vi "PH_BeamlineController.set wanted Path to World.vi"(0 "VI in":refnum<vi>, 5 "error in (no error)":errorcluster) -> (14 "VI out":refnum<vi>, 19 "error out":errorcluster)   [LabVIEW 2014, in "PH_BeamlineController.lvlib"]
uses:
  PH_BeamlineController.lvlib
  PH_SystemInformation/PH_SystemInformationEnabling State.ctl
  PH_Beamline/PH_Beamline.6P Switch Instances.ctl
  PH_Beamline/PH_Beamline.Black Box Instances.ctl
  PH_StatusHandler/PH_StatusHandler.Status.ctl
  PH_BeamlineController.Targets.ctl
  PH_BeamlineController.PA DP Targets.ctl
  PH_Beamline/PH_Beamline.Switch Instances.ctl
  PH_Beamline/PH_Beamline.lvlib
  PH_BlackBox/PH_BlackBox.lvlib
  PH_SystemInformation/PH_SystemInformation.lvlib
  PH_Sixpack_Switch/PH_Sixpack_Switch.lvlib
  PH_Switch/PH_Switch.lvlib
  PH_StatusHandler/PH_StatusHandler.lvlib
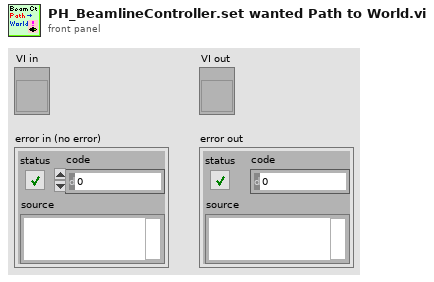
[diagram p1: front panel]
types:
  T1 = typedef "PH_Beamline.lvlib/PH_Beamline.Black Box Instances.ctl" = string
  T2 = typedef "PH_BeamlineController.lvlib/PH_BeamlineController.PA DP Targets.ctl" = enum16{"None", "Dump PA Delayed Beam", "Dump PA Undelayed Beam", "Dumps PA Delayed and Undelayed Beam"}
  T3 = typedef "PH_BeamlineController.lvlib/PH_BeamlineController.Targets.ctl" = enum16{"None", "PreAmp", "Dump Exp Laserlab", "Exp Laserlab", "Calorimeter", "Dump Exp Laserbay", "Exp Laserbay", "Dump Exp Z6", "Exp Z6"}
  T4 = typedef "PH_StatusHandler.lvlib/PH_StatusHandler.Status.ctl" = i16
  T5 = typedef "PH_SystemInformation.lvlib/PH_SystemInformationEnabling State.ctl" = i32
  T6 = enum16{"Laser", "PreAmp", "MainAmp", "Exp 1", "Exp 2", "Exp 3", "Exp 4"}
  T7 = typedef "PH_Beamline.lvlib/PH_Beamline.6P Switch Instances.ctl" = string
  T8 = typedef "PH_BeamlineController.lvlib/PH_BeamlineController.Sources.ctl" = enum16{"None", "YLF", "fs-Frontend", "ns-Frontend", "YLF and ns-Frontend", "fs- and ns-Frontend"}
  T9 = typedef "PH_Beamline.lvlib/PH_Beamline.Switch Instances.ctl" = string
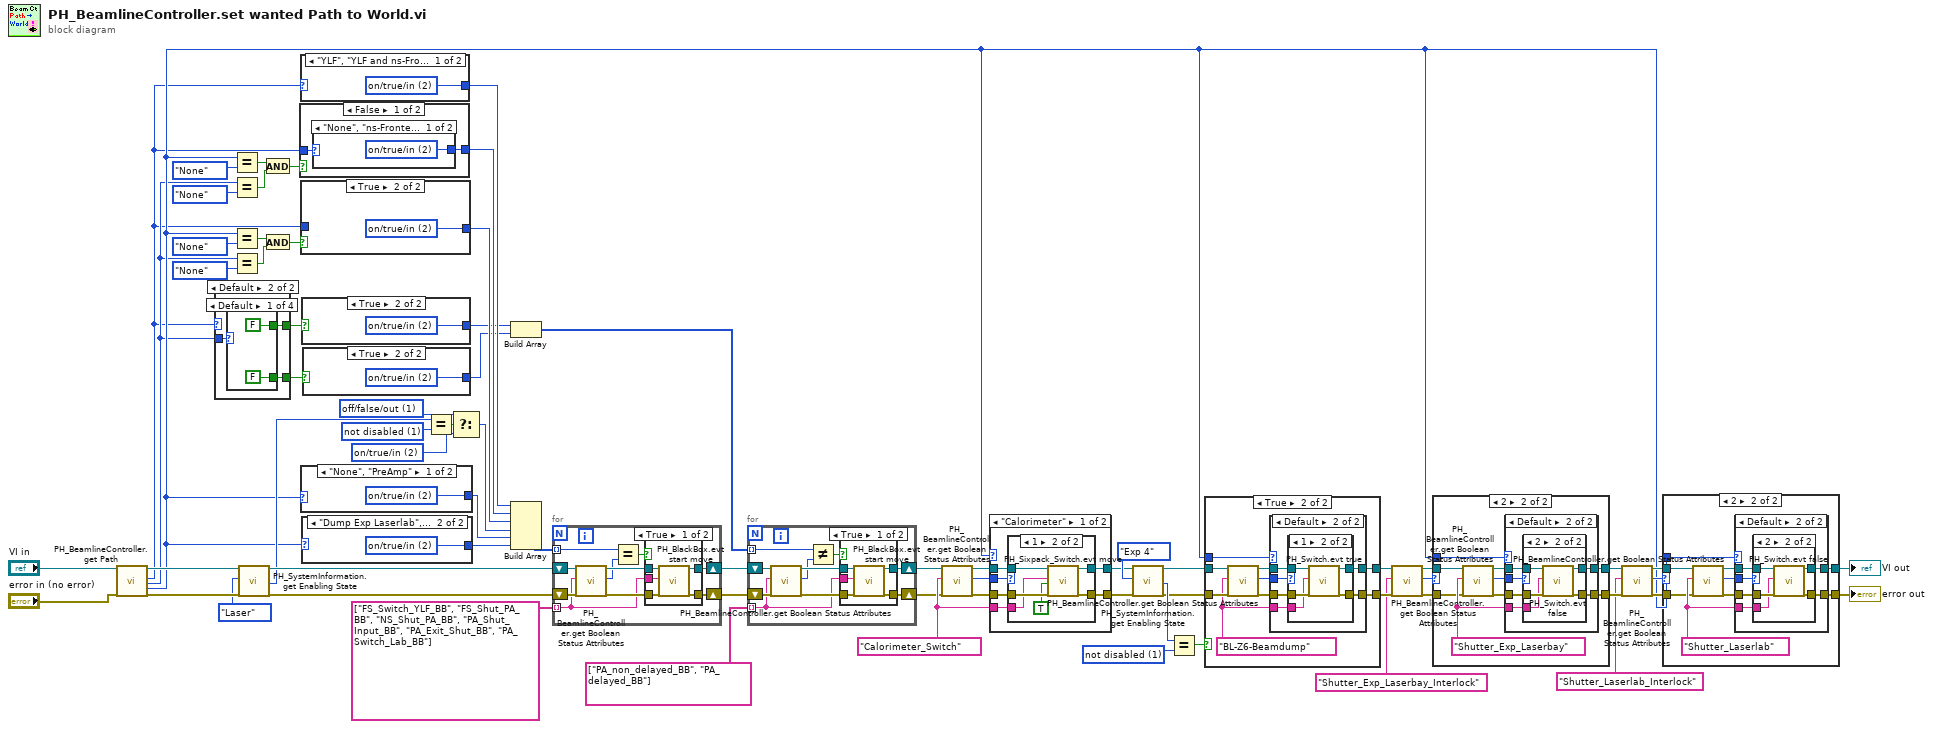
[diagram p0: block diagram]
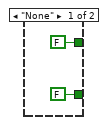
[diagram p3: hidden frame]
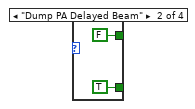
[diagram p4: hidden frame]
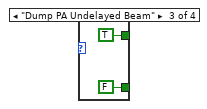
[diagram p5: hidden frame]
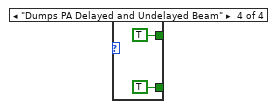
[diagram p6: hidden frame]
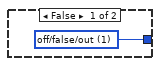
[diagram p7: hidden frame]
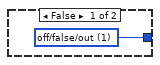
[diagram p8: hidden frame]
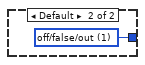
[diagram p10: hidden frame]
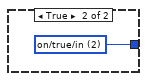
[diagram p11: hidden frame]
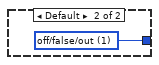
[diagram p12: hidden frame]
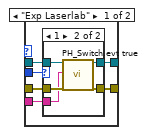
[diagram p14: hidden frame]
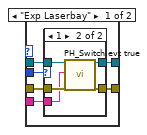
[diagram p18: hidden frame]
diagram:
  w44 = T4 2 items=["no info", "off/false/out", "on/true/in", "Failure", "Alarm", "Status 1", "Status 2", "Status 3"] ("f")
  w45 = T4 1 items=["no info", "off/false/out", "on/true/in", "Failure", "Alarm", "Status 1", "Status 2", "Status 3"] ("y")
  w67 = T5 1 items=["no info", "not disabled", "disabled"] ("x")
  w40 = T7 "Calorimeter_Switch" ("6P Switch Instances")
  w68 = T5 1 items=["no info", "not disabled", "disabled"] ("x")
  n1 = call "PH_BeamlineController.get Path.vi"("VI in"="VI in", "error in (no error)"="error in (no error)") -> ("VI out"=w29:refnum<vi>, "Path: Source"=w9:T8, "Path:  PA DP Targets"=w12:T2, "Path: Target"=w17:T3, "error out"=w27:errorcluster)  [unwired: 12 in, 1 out]
  n2 = case shown="Default" w9 {
    tunnel: w12 -> [_ w74]
    tunnel: [FALSE w73] -> w11
    tunnel: [FALSE w72] -> w10
    frame "None" {
    }
    frame Default {
      n3 = case shown="Default" w74 {
        tunnel: [FALSE TRUE FALSE TRUE] -> w73
        tunnel: [FALSE FALSE TRUE TRUE] -> w72
        frame Default {
        }
        frame "Dump PA Delayed Beam" {
        }
        frame "Dump PA Undelayed Beam" {
        }
        frame "Dumps PA Delayed and Undelayed Beam" {
        }
      }
    }
  }
  n4 = Equal?(x=w17, y=PH_BeamlineController.Targets."None") -> (x = y?=w23:bool)
  n5 = Equal?(x=w12, y=PH_BeamlineController.PA_DP_Targets."None") -> (x = y?=w20:bool)
  n6 = Equal?(x=w17, y=PH_BeamlineController.Targets."None") -> (x = y?=w16:bool)
  n7 = Equal?(x=w12, y=PH_BeamlineController.PA_DP_Targets."None") -> (x = y?=w18:bool)
  n8 = call "PH_SystemInformation.get Enabling State.vi"("i ref in"=w29, "Wanted State"=T6."Laser", "error in (no error)"=w27) -> ("i ref out"=w28:refnum<vi>, "Enabling State"=w25:T5, "error out"=w26:errorcluster)  [unwired: 14 in]
  n9 = And(x=w23, y=w20) -> (x .and. y?=w21:bool)
  n10 = And(x=w16, y=w18) -> (x .and. y?=w14:bool)
  n11 = case shown="False" w21 {
    tunnel: w9 -> [w84 _]
    tunnel: [w83 w87] -> w48
    frame False {
      n12 = case shown="\"None\", \"ns-Frontend\"" w84 {
        tunnel: [w85 w86] -> w83
        frame "None", "ns-Frontend" {
          w85 = T4 2 items=["no info", "off/false/out", "on/true/in", "Failure", "Alarm", "Status 1", "Status 2", "Status 3"] ("y")
        }
        frame Default {
          w86 = T4 1 items=["no info", "off/false/out", "on/true/in", "Failure", "Alarm", "Status 1", "Status 2", "Status 3"] ("y")
        }
      }
    }
    frame True {
      w87 = T4 2 items=["no info", "off/false/out", "on/true/in", "Failure", "Alarm", "Status 1", "Status 2", "Status 3"] ("y")
    }
  }
  n13 = case shown="\"YLF\", \"YLF and ns-Frontend\"" w9 {
    tunnel: [w88 w89] -> w51
    frame "YLF", "YLF and ns-Frontend" {
      w88 = T4 2 items=["no info", "off/false/out", "on/true/in", "Failure", "Alarm", "Status 1", "Status 2", "Status 3"] ("y")
    }
    frame Default {
      w89 = T4 1 items=["no info", "off/false/out", "on/true/in", "Failure", "Alarm", "Status 1", "Status 2", "Status 3"] ("y")
    }
  }
  n14 = case shown="True" w14 {
    tunnel: w9 -> [w91 _]
    tunnel: [w90 w94] -> w47
    frame False {
      n15 = case shown="\"None\"..\"fs-Frontend\"" w91 {
        tunnel: [w92 w93] -> w90
        frame "None".."fs-Frontend" {
          w92 = T4 2 items=["no info", "off/false/out", "on/true/in", "Failure", "Alarm", "Status 1", "Status 2", "Status 3"] ("y")
        }
        frame Default {
          w93 = T4 1 items=["no info", "off/false/out", "on/true/in", "Failure", "Alarm", "Status 1", "Status 2", "Status 3"] ("y")
        }
      }
    }
    frame True {
      w94 = T4 2 items=["no info", "off/false/out", "on/true/in", "Failure", "Alarm", "Status 1", "Status 2", "Status 3"] ("y")
    }
  }
  n16 = case shown="\"None\", \"PreAmp\"" w17 {
    tunnel: [w95 w96] -> w42
    frame "None", "PreAmp" {
      w95 = T4 2 items=["no info", "off/false/out", "on/true/in", "Failure", "Alarm", "Status 1", "Status 2", "Status 3"] ("y")
    }
    frame Default {
      w96 = T4 1 items=["no info", "off/false/out", "on/true/in", "Failure", "Alarm", "Status 1", "Status 2", "Status 3"] ("y")
    }
  }
  n17 = case shown="True" w10 {
    tunnel: [w97 w98] -> w3
    frame False {
      w97 = T4 1 items=["no info", "off/false/out", "on/true/in", "Failure", "Alarm", "Status 1", "Status 2", "Status 3"] ("y")
    }
    frame True {
      w98 = T4 2 items=["no info", "off/false/out", "on/true/in", "Failure", "Alarm", "Status 1", "Status 2", "Status 3"] ("y")
    }
  }
  n18 = case shown="\"Dump Exp Laserlab\", \"Exp Laserlab\"" w17 {
    tunnel: [w99 w100] -> w41
    frame Default {
      w99 = T4 1 items=["no info", "off/false/out", "on/true/in", "Failure", "Alarm", "Status 1", "Status 2", "Status 3"] ("y")
    }
    frame "Dump Exp Laserlab", "Exp Laserlab" {
      w100 = T4 2 items=["no info", "off/false/out", "on/true/in", "Failure", "Alarm", "Status 1", "Status 2", "Status 3"] ("y")
    }
  }
  n19 = case shown="True" w11 {
    tunnel: [w101 w102] -> w2
    frame False {
      w101 = T4 1 items=["no info", "off/false/out", "on/true/in", "Failure", "Alarm", "Status 1", "Status 2", "Status 3"] ("y")
    }
    frame True {
      w102 = T4 2 items=["no info", "off/false/out", "on/true/in", "Failure", "Alarm", "Status 1", "Status 2", "Status 3"] ("y")
    }
  }
  n20 = Equal?(x=w25, y=w68) -> (x = y?=w46:bool)
  n21 = Select(t=w45, s=w46, f=w44) -> (s? t:f=w43:T4)
  n22 = Build Array(w3, w2) -> (w1:T4[])
  n23 = Build Array(w51, w48, w47, w43, w42, w41) -> (w49:T4[])
  n24 = for {
    tunnel: w49 -> [w112] mode=indexing
    shift-right: [w105] -> w8
    shift-left: w26 -> [w108]
    shift-right: [w106] -> w7
    shift-left: w28 -> [w107]
    tunnel: T1[] ["FS_Switch_YLF_BB", "FS_Shut_PA_BB", "NS_Shut_PA_BB", "PA_Shut_Input_BB", "PA_Exit_Shut_BB", "PA_Switch_Lab_BB"] -> [w103] mode=indexing
    n25 = call "PH_BeamlineController.get Boolean Status Attributes.vi"("VI in"=w107, "Name"=w103, "error in (no error)"=w108) -> ("VI out"=w110:refnum<vi>, "Status"=w104:T4, "error out"=w109:errorcluster)  [unwired: 11 in, 3 out]
    n26 = Equal?(x=w112, y=w104) -> (x = y?=w111:bool)
    n27 = case shown="True" w111 {
      tunnel: w109 -> [w113 w118]
      tunnel: [w117 w118] -> w105
      tunnel: w110 -> [w114 w119]
      tunnel: [w116 w119] -> w106
      tunnel: w103 -> [w115 _]
      frame True {
        n28 = call "PH_BlackBox.evt start move.vi"("i ref in"=w114, "Instance"=w115, "error in (no error)"=w113) -> ("i ref out"=w116:refnum<vi>, "error out"=w117:errorcluster)  [unwired: 15 in]
      }
      frame False {
      }
    }
  }
  n29 = for {
    tunnel: w1 -> [w129] mode=indexing
    shift-right: [w122] -> w5
    shift-left: w8 -> [w125]
    shift-right: [w123] -> w6
    shift-left: w7 -> [w124]
    tunnel: T1[] ["PA_non_delayed_BB", "PA_delayed_BB"] -> [w120] mode=indexing
    n30 = call "PH_BeamlineController.get Boolean Status Attributes.vi"("VI in"=w124, "Name"=w120, "error in (no error)"=w125) -> ("VI out"=w127:refnum<vi>, "Status"=w121:T4, "error out"=w126:errorcluster)  [unwired: 11 in, 3 out]
    n31 = Not Equal?(x=w129, y=w121) -> (x != y?=w128:bool)
    n32 = case shown="True" w128 {
      tunnel: w126 -> [w130 w135]
      tunnel: [w134 w135] -> w122
      tunnel: w127 -> [w131 w136]
      tunnel: [w133 w136] -> w123
      tunnel: w120 -> [w132 _]
      frame True {
        n33 = call "PH_BlackBox.evt start move.vi"("i ref in"=w131, "Instance"=w132, "error in (no error)"=w130) -> ("i ref out"=w133:refnum<vi>, "error out"=w134:errorcluster)  [unwired: 15 in]
      }
      frame False {
      }
    }
  }
  n34 = call "PH_BeamlineController.get Boolean Status Attributes.vi"("VI in"=w6, "Name"=w40, "error in (no error)"=w5) -> ("VI out"=w39:refnum<vi>, "Status"=w37:T4, "error out"=w38:errorcluster)  [unwired: 11 in, 3 out]
  n35 = case shown="\"Calorimeter\"" w17 {
    tunnel: w39 -> [w142 w156]
    tunnel: [w141 w155] -> w34
    tunnel: w38 -> [w140 w154]
    tunnel: [w139 w153] -> w35
    tunnel: w37 -> [w138 w152]
    tunnel: w40 -> [w137 w151]
    frame "Calorimeter" {
      n36 = case shown="1" w138 {
        tunnel: w142 -> [w144 w150]
        tunnel: [w144 w149] -> w141
        tunnel: w140 -> [w143 w148]
        tunnel: [w143 w147] -> w139
        tunnel: w137 -> [_ w145]
        frame Default {
        }
        frame 1 {
          n37 = call "PH_Sixpack_Switch.evt move.vi"("i ref in"=w150, "Instance"=w145, "Move"=TRUE, "error in (no error)"=w148) -> ("i ref out"=w149:refnum<vi>, "error out"=w147:errorcluster)  [unwired: 14 in]
        }
      }
    }
    frame Default {
      n38 = case shown="2" w152 {
        tunnel: w156 -> [w158 w164]
        tunnel: [w158 w163] -> w155
        tunnel: w154 -> [w157 w162]
        tunnel: [w157 w161] -> w153
        tunnel: w151 -> [_ w159]
        frame Default {
        }
        frame 2 {
          n39 = call "PH_Sixpack_Switch.evt move.vi"("i ref in"=w164, "Instance"=w159, "Move"=TRUE, "error in (no error)"=w162) -> ("i ref out"=w163:refnum<vi>, "error out"=w161:errorcluster)  [unwired: 14 in]
        }
      }
    }
  }
  n40 = call "PH_SystemInformation.get Enabling State.vi"("i ref in"=w34, "Wanted State"=T6."Exp 4", "error in (no error)"=w35) -> ("i ref out"=w33:refnum<vi>, "Enabling State"=w36:T5, "error out"=w32:errorcluster)  [unwired: 14 in]
  n41 = Equal?(x=w36, y=w67) -> (x = y?=w66:bool)
  n42 = case shown="True" w66 {
    tunnel: [w166 w172] -> w64
    tunnel: w33 -> [w166 w171]
    tunnel: [w165 w170] -> w62
    tunnel: w32 -> [w165 w169]
    tunnel: w17 -> [_ w168]
    frame False {
    }
    frame True {
      w167 = T9 "BL-Z6-Beamdump" ("Switch Instances")
      n43 = call "PH_BeamlineController.get Boolean Status Attributes.vi"("VI in"=w171, "Name"=w167, "error in (no error)"=w169) -> ("VI out"=w173:refnum<vi>, "Status"=w175:T4, "error out"=w174:errorcluster)  [unwired: 11 in, 3 out]
      n44 = case shown="Default" w168 {
        tunnel: w173 -> [w181 w194]
        tunnel: [w180 w193] -> w172
        tunnel: w174 -> [w179 w192]
        tunnel: [w178 w191] -> w170
        tunnel: w175 -> [w177 w190]
        tunnel: w167 -> [w176 w189]
        frame "Exp Z6" {
          n45 = case shown="2" w177 {
            tunnel: w181 -> [w183 w188]
            tunnel: [w183 w187] -> w180
            tunnel: w179 -> [w182 w186]
            tunnel: [w182 w185] -> w178
            tunnel: w176 -> [_ w184]
            frame Default {
            }
            frame 2 {
              n46 = call "PH_Switch.evt false.vi"("i ref in"=w188, "Instance"=w184, "error in (no error)"=w186) -> ("i ref out"=w187:refnum<vi>, "error out"=w185:errorcluster)  [unwired: 15 in]
            }
          }
        }
        frame Default {
          n47 = case shown="1" w190 {
            tunnel: w194 -> [w196 w201]
            tunnel: [w196 w200] -> w193
            tunnel: w192 -> [w195 w199]
            tunnel: [w195 w198] -> w191
            tunnel: w189 -> [_ w197]
            frame Default {
            }
            frame 1 {
              n48 = call "PH_Switch.evt true.vi"("i ref in"=w201, "Instance"=w197, "error in (no error)"=w199) -> ("i ref out"=w200:refnum<vi>, "error out"=w198:errorcluster)  [unwired: 15 in]
            }
          }
        }
      }
    }
  }
  n49 = call "PH_BeamlineController.get Boolean Status Attributes.vi"("VI in"=w64, "Name"="Shutter_Exp_Laserbay_Interlock" ("Instance PA Backreflection"), "error in (no error)"=w62) -> ("VI out"=w65:refnum<vi>, "Status"=w61:T4, "error out"=w63:errorcluster)  [unwired: 11 in, 3 out]
  n50 = case shown="2" w61 {
    tunnel: [w203 w208] -> w55
    tunnel: w65 -> [w203 w207]
    tunnel: [w202 w206] -> w56
    tunnel: w63 -> [w202 w205]
    tunnel: w17 -> [_ w204]
    frame Default {
    }
    frame 2 {
      w209 = T9 "Shutter_Exp_Laserbay" ("Switch Instances")
      n51 = call "PH_BeamlineController.get Boolean Status Attributes.vi"("VI in"=w207, "Name"=w209, "error in (no error)"=w205) -> ("VI out"=w210:refnum<vi>, "Status"=w212:T4, "error out"=w211:errorcluster)  [unwired: 11 in, 3 out]
      n52 = case shown="Default" w204 {
        tunnel: w210 -> [w218 w231]
        tunnel: [w217 w230] -> w208
        tunnel: w211 -> [w216 w229]
        tunnel: [w215 w228] -> w206
        tunnel: w212 -> [w214 w227]
        tunnel: w209 -> [w213 w226]
        frame "Exp Laserbay" {
          n53 = case shown="1" w214 {
            tunnel: w218 -> [w220 w225]
            tunnel: [w220 w224] -> w217
            tunnel: w216 -> [w219 w223]
            tunnel: [w219 w222] -> w215
            tunnel: w213 -> [_ w221]
            frame Default {
            }
            frame 1 {
              n54 = call "PH_Switch.evt true.vi"("i ref in"=w225, "Instance"=w221, "error in (no error)"=w223) -> ("i ref out"=w224:refnum<vi>, "error out"=w222:errorcluster)  [unwired: 15 in]
            }
          }
        }
        frame Default {
          n55 = case shown="2" w227 {
            tunnel: w231 -> [w233 w238]
            tunnel: [w233 w237] -> w230
            tunnel: w229 -> [w232 w236]
            tunnel: [w232 w235] -> w228
            tunnel: w226 -> [_ w234]
            frame Default {
            }
            frame 2 {
              n56 = call "PH_Switch.evt false.vi"("i ref in"=w238, "Instance"=w234, "error in (no error)"=w236) -> ("i ref out"=w237:refnum<vi>, "error out"=w235:errorcluster)  [unwired: 15 in]
            }
          }
        }
      }
    }
  }
  n57 = call "PH_BeamlineController.get Boolean Status Attributes.vi"("VI in"=w55, "Name"="Shutter_Laserlab_Interlock" ("Instance PA Backreflection"), "error in (no error)"=w56) -> ("VI out"=w59:refnum<vi>, "Status"=w57:T4, "error out"=w58:errorcluster)  [unwired: 11 in, 3 out]
  n58 = case shown="2" w57 {
    tunnel: [w240 w245] -> w53
    tunnel: w59 -> [w240 w244]
    tunnel: [w239 w243] -> w52
    tunnel: w58 -> [w239 w242]
    tunnel: w17 -> [_ w241]
    frame Default {
    }
    frame 2 {
      w246 = T9 "Shutter_Laserlab" ("Switch Instances")
      n59 = call "PH_BeamlineController.get Boolean Status Attributes.vi"("VI in"=w244, "Name"=w246, "error in (no error)"=w242) -> ("VI out"=w247:refnum<vi>, "Status"=w249:T4, "error out"=w248:errorcluster)  [unwired: 11 in, 3 out]
      n60 = case shown="Default" w241 {
        tunnel: w247 -> [w255 w268]
        tunnel: [w254 w267] -> w245
        tunnel: w248 -> [w253 w266]
        tunnel: [w252 w265] -> w243
        tunnel: w249 -> [w251 w264]
        tunnel: w246 -> [w250 w263]
        frame "Exp Laserlab" {
          n61 = case shown="1" w251 {
            tunnel: w255 -> [w257 w262]
            tunnel: [w257 w261] -> w254
            tunnel: w253 -> [w256 w260]
            tunnel: [w256 w259] -> w252
            tunnel: w250 -> [_ w258]
            frame Default {
            }
            frame 1 {
              n62 = call "PH_Switch.evt true.vi"("i ref in"=w262, "Instance"=w258, "error in (no error)"=w260) -> ("i ref out"=w261:refnum<vi>, "error out"=w259:errorcluster)  [unwired: 15 in]
            }
          }
        }
        frame Default {
          n63 = case shown="2" w264 {
            tunnel: w268 -> [w270 w275]
            tunnel: [w270 w274] -> w267
            tunnel: w266 -> [w269 w273]
            tunnel: [w269 w272] -> w265
            tunnel: w263 -> [_ w271]
            frame Default {
            }
            frame 2 {
              n64 = call "PH_Switch.evt false.vi"("i ref in"=w275, "Instance"=w271, "error in (no error)"=w273) -> ("i ref out"=w274:refnum<vi>, "error out"=w272:errorcluster)  [unwired: 15 in]
            }
          }
        }
      }
    }
  }
  "VI out" <- w53
  "error out" <- w52
